vi "Laser_Ethernet_Init.vi"(8 "error in (no error)":errorcluster, 10 "Name":string, 11 "object in":refnum<class "Laser_Ethernet.lvclass">) -> (0 "error out":errorcluster, 3 "object out":refnum<class "Laser_Ethernet.lvclass">)   [LabVIEW 2023, in "Laser_Ethernet.lvclass"]
uses:
  Laser_Ethernet.lvclass
  Laser_Ethernet.lvclass/Laser_Ethernet.ctl
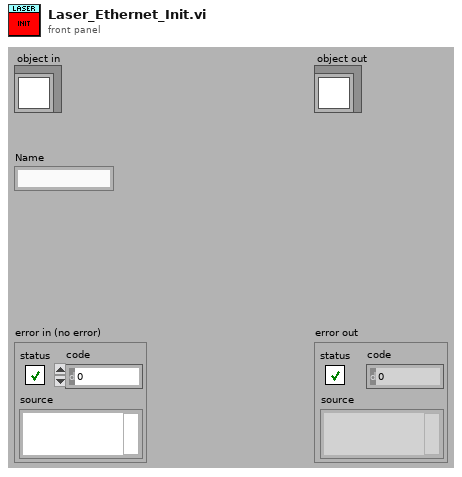
[diagram p1: front panel]
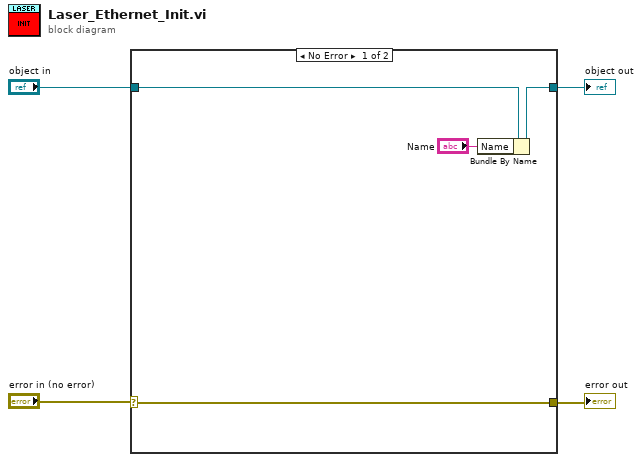
[diagram p0: block diagram]
diagram:
  n1 = case shown="No Error" "error in (no error)" {
    selector: "error in (no error)" -> [w6 w9]
    tunnel: "object in" -> [w8 w10]
    tunnel: [w7 w10] -> w3
    tunnel: [w6 w9] -> w1
    frame No Error {
      n2 = Bundle By Name(cluster=w8, "Name"="Name") -> (w7:refnum<class "Laser_Ethernet.lvclass">)
    }
    frame Error {
    }
  }
  "object out" <- w3
  "error out" <- w1
